vi "Format File Property.vi"(8 "Error In":errorcluster, 9 "File Property Value":string, 10 "File Property Name":string, 11 "String in":string) -> (0 "Error Out":errorcluster, 3 "String out":string)   [LabVIEW 2014]
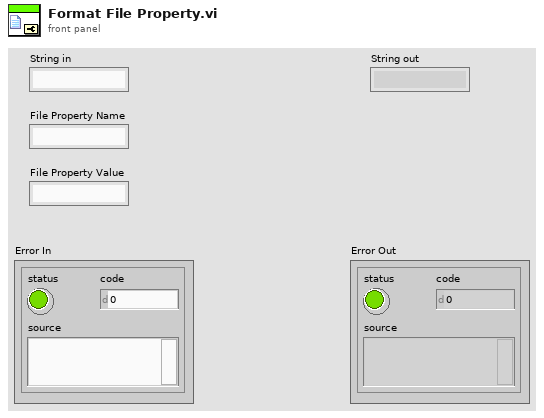
[diagram p1: front panel]
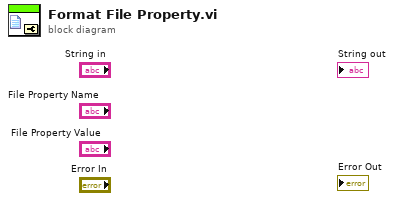
[diagram p0: block diagram]
diagram:
